vi "1-Exp (X) Gaussian Fit.vi"(6 "Weighted Fit":T1, 8 "Error In":errorcluster, 9 "Plot Name":string, 10 "Y Array":dbl[](array[numeric]), 11 "X Array":dbl[](array[numeric])) -> (0 "Error Out":errorcluster, 1 "Fit Result String":string, 2 "Fitted Y Array":dbl[](array[numeric]), 3 "X Array":dbl[](array[numeric]))   [LabVIEW 2021, in "Fits.lvlib"]
doc: "Extract IRF from provided decay and time constant"
uses:
  Fits.lvlib
  <vilib>/Analysis/NI_AALPro.lvlib
  LM model function and gradient (Gaussian (X) 1-Exp).vi
  <vilib>/Analysis/6fits.llb/Curve Fitting Criteria.ctl
  Error/Error.lvlib
  IRF(X)PSED/Fit Weights Type v2.ctl
panel:
  out "best fit parameters":dbl[](array[numeric])
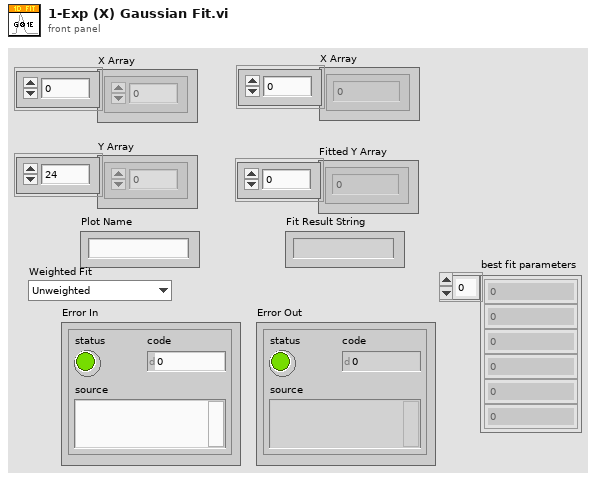
[diagram p1: front panel]
types:
  T1 = typedef "Fits.lvlib/Fit Weights Type v2.ctl" = enum16{"Unweighted", "1/Variance (Neyman)", "1/Variance (Pearson)", "Best of All"}
  T2 = cluster{"parameter minimum":dbl[], "parameter maximum":dbl[]}
  T3 = cluster{"amp min":dbl, "amp max":dbl, "center min":dbl, "center max":dbl, "deviation min":dbl, "deviation max":dbl, "offset min":dbl, "offset max":dbl}
  T4 = cluster{"initial amplitude":dbl, "initial center":dbl, "initial standard deviation":dbl, "offset":dbl}
  T5 = typedef "NI_AALPro.lvlib/Curve Fitting Criteria.ctl" = u16
  T6 = typedef "Fits.lvlib/Gaussian Fit Parameters.ctl" = cluster{"Center":dbl, "Baseline":dbl, "Amplitude":dbl, "Standard Deviation":dbl}
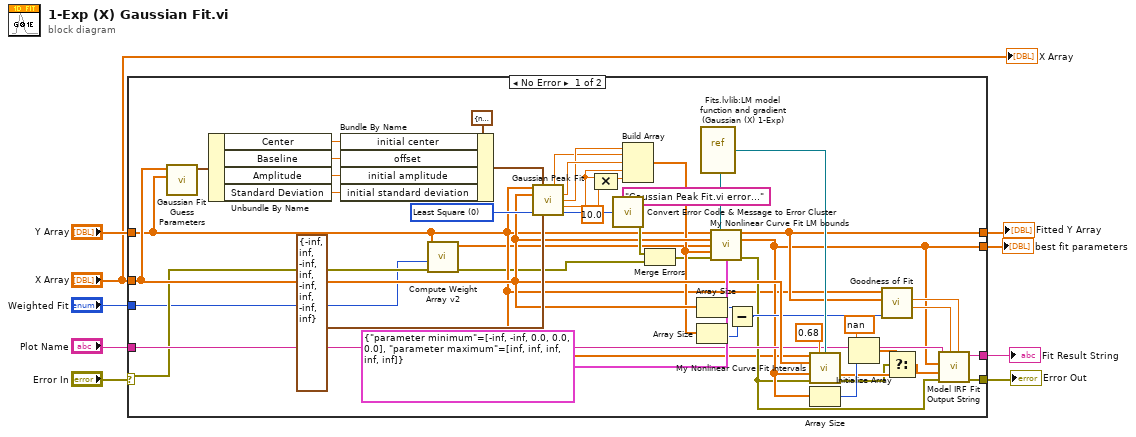
[diagram p0: block diagram]
diagram:
  n1 = case shown="No Error" "Error In" {
    selector: "Error In" -> [w13 w56]
    tunnel: "Y Array" -> [w15 _]
    tunnel: [w37 w56] -> w8
    tunnel: [w26 _] -> w7
    tunnel: [w28 _] -> w6
    tunnel: "X Array" -> [w34 _]
    tunnel: [w30 _] -> w5
    tunnel: "Plot Name" -> [w29 _]
    tunnel: "Weighted Fit" -> [w12 _]
    frame No Error {
      w43 = T5 0 items=["Least Square", "Least Absolute Residual", "Bisquare"] ("method")
      n2 = call "Gaussian Fit Guess Parameters.vi"("Y Array"=w15, "X Array"=w34) -> ("Gaussian Fit Parameters"=w48:T6)  [unwired: 9 in]
      n3 = Unbundle By Name(w48) -> ("Center"=w54:dbl, "Baseline"=w53:dbl, "Amplitude"=w52:dbl, "Standard Deviation"=w51:dbl)
      n4 = Bundle By Name(cluster=T4 {"initial amplitude"=nan, "initial center"=nan, "initial standard deviation"=nan, "offset"=nan} ("initial guess"), "initial center"=w54, "offset"=w53, "initial amplitude"=w52, "initial standard deviation"=w51) -> (w50:T4)
      n5 = call "Compute Weight Array v2.vi"("Error In"=w13, "Weighted Fit"=w12, "Data Array"=w15) -> ("Error Out"=w10:errorcluster, "Weight Array"=w14:dbl[])  [unwired: 7 in]
      n6 = call <vilib>:"Gaussian Peak Fit.vi"("Y"=w15, "initial guess"=w50, "X"=w34, "method"=w43, "parameter bounds"=T3 {"amp min"=-inf, "amp max"=inf, "center min"=-inf, "center max"=inf, "deviation min"=-inf, "deviation max"=inf, "offset min"=-inf, "offset max"=inf}) -> ("offset"=w44:dbl, "amplitude"=w47:dbl, "center"=w46:dbl, "standard deviation"=w17:dbl, "error"=w42:i32)  [unwired: 4 in, 2 out]
      n7 = Compound Arithmetic op=MULTIPLY(w17, 10.0 ("value")) -> (w18:dbl)
      n8 = call "Convert Error Code & Message to Error Cluster.vi"("Error Code (no error: 0)"=w42, "Error Message"="Gaussian Peak Fit.vi error...") -> ("Error Out"=w40:errorcluster)
      n9 = Build Array(w46, w44, w47, w17, w18) -> (w33:dbl[])
      n10 = Merge Errors(w40, w10) -> (w11:errorcluster)
      n11 = Array Size(array=w34) -> (size(s)=w36:i32)
      n12 = Array Size(array=w33) -> (size(s)=w35:i32)
      n13 = vi-ref "Fits.lvlib:LM model function and gradient (Gaussian (X) 1-Exp).vi"() -> (w39:refnum<vi>)
      n14 = call "My Nonlinear Curve Fit LM bounds.vi"("Y"=w15, "f(x,a)"=w39, "X"=w34, "Weight"=w14, "initial parameters"=w33, "error in (no error)"=w11, "parameter bounds"=T2 {"parameter minimum"=[-inf, -inf, 0.0, 0.0, 0.0], "parameter maximum"=[inf, inf, inf, inf, inf]}) -> ("best nonlinear fit"=w28:dbl[], "best fit parameters"=w26:dbl[], "error out"=w19:errorcluster)  [unwired: 3 in, 3 out]
      n15 = Subtract(x=w36, y=w35) -> (x-y=w27:i32)
      n16 = call "My Nonlinear Curve Fit Intervals.vi"("Y"=w15, "confidence level"=0.68, "f(x,a)"=w39, "X"=w34, "best fit parameters"=w26, "error in (no error)"=w19) -> ("delta best fit parameters"=w22:dbl[], "error out"=w21:errorcluster)  [unwired: 8 in]
      n17 = Array Size(array=w26) -> (size(s)=w25:i32)
      n18 = Initialize Array(nan ("element"), w25) -> (w23:dbl[])
      n19 = call <vilib>:"Goodness of Fit.vi"("degree of freedom"=w27, "Best Fit"=w28, "Y"=w15) -> ("RMSE"=w31:dbl, "R-square"=w32:dbl)  [unwired: 5 in, 2 out]
      n20 = Select(t=w23, s=w21, f=w22) -> (s? t:f=w20:dbl[])
      n21 = call "Model IRF Fit Output String.vi"("R^2"=w32, "Reduced Chi^2"=w31, "Error In"=w19, "Delta Best Fit Parameters"=w20, "Best Fit Parameters"=w26, "Plot Name"=w29) -> ("Error Out"=w37:errorcluster, "Fit Output Message"=w30:string)  [unwired: 4 in]
    }
    frame Error {
    }
  }
  "Fitted Y Array" <- w6
  "Error Out" <- w8
  "best fit parameters" <- w7
  "Fit Result String" <- w5
  "X Array" <- "X Array"
